vi "Configure Coupling.vi"(8 "error in (no error)":errorcluster, 10 "External Control Coupling (0:AC)":u16(ring) items=["AC", "DC", "AC+DC"], 11 "VISA resource name":refnum<visa-resource-name>) -> (0 "error out":errorcluster, 3 "VISA resource name out":refnum<visa-resource-name>)   [LabVIEW 2015, in "BK Precision 983X Series.lvlib"]
doc: "Configures the output coupling mode for normal operation, digital I/O and external voltage control."
uses:
  <instrlib>/BK Precision 983X Series/BK Precision 983X Series.lvlib
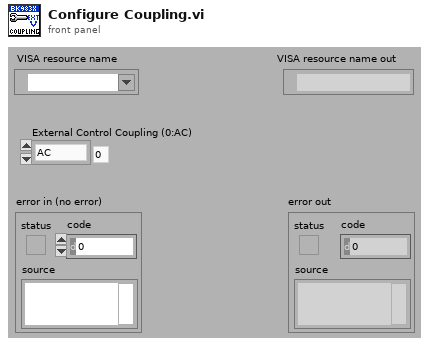
[diagram p1: front panel]
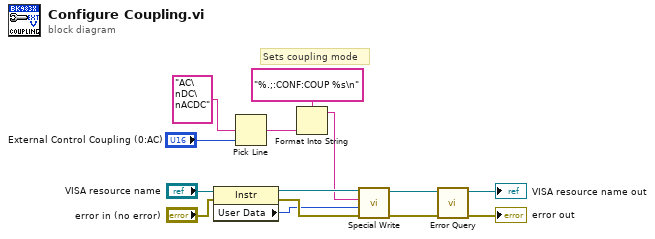
[diagram p0: block diagram]
diagram:
  # "Sets coupling mode"
  n1 = property class="Instr"(reference="VISA resource name", error in="error in (no error)") -> (reference out=w4:refnum<visa-resource-name>, error out=w6:errorcluster, "User Data"=w5:u32)
  n2 = Pick Line(multi-line string="AC\nDC\nACDC", line index="External Control Coupling (0:AC)") -> (output string=w2:string)  [unwired: 1 in]
  n3 = Format Into String(format string="%.;:CONF:COUP %s\n" ("string (\"\")"), w2) -> (resulting string=w1:string)  [unwired: 2 in, 1 out]
  n4 = call <instrlib>:"Special Write.vi"("error in (no error)"=w6, "Delay (0 ms)"=w5, "Input String"=w1, "VISA resource name"=w4) -> ("error out"=w9:errorcluster, "VISA resource name out"=w10:refnum<visa-resource-name>)  [unwired: 6 in]
  n5 = call <instrlib>:"Error Query.vi"("error in (no error)"=w9, "VISA resource name"=w10) -> ("error out"=→"error out":errorcluster, "VISA resource name out"=→"VISA resource name out":refnum<visa-resource-name>)  [unwired: 6 in, 2 out]
